vi "VI Tree.vi"   [LabVIEW 2017, in "Keithley 3390.lvlib"]
doc: "This is the instrument driver for the <INSTRUMENT NAME>. The VI Tree displays all the user-callable VIs of the instrument driver in an organized table."
uses:
  Keithley 3390.lvlib
  Configure/Configure Modulation (Amplitude).vi
  Configure/Low Level/Configure Voltage (Amplitude).vi
  Configure/Low Level/Configure Pulse (Period).vi
  Configure/Low Level/Configure Modulation Low Level (AM Depth).vi
  Configure/Configure Waveform (Sine).vi
panel:
  # "(c) 2008 Keithley Instruments, Inc..  ALL RIGHTS RESERVED."
  # "SEE DIAGRAM\nFOR VI TREE."
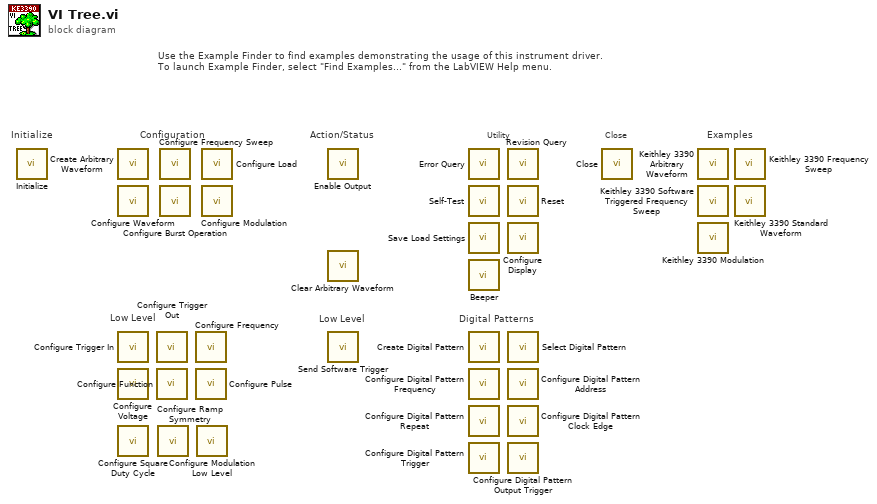
[diagram p0: block diagram]
diagram:
  # "Examples"
  # "Digital Patterns"
  # "Low Level"
  # "Low Level"
  # "Use the Example Finder to find examples demonstrating the usage of this instrument driver.\nTo launch Example Finder, select \"Find Examples...\" from the LabVIEW Help menu."
  # "Configuration"
  # "Utility"
  # "Action/Status"
  # "Close"
  # "Initialize"
  n1 = call "Initialize.vi"() -> ()  [unwired: 10 in, 2 out]
  n2 = call "Create Arbitrary Waveform.vi"() -> ()  [unwired: 10 in, 2 out]
  n3 = call-poly "Configure Waveform.vi"() -> ()  [unwired: 14 in, 2 out]
  n4 = call "Configure Trigger In.vi"() -> ()  [unwired: 10 in, 2 out]
  n5 = call-poly "Configure Voltage.vi"() -> ()  [unwired: 10 in, 2 out]
  n6 = call "Configure Square Duty Cycle.vi"() -> ()  [unwired: 10 in, 2 out]
  n7 = call "Configure Trigger Out.vi"() -> ()  [unwired: 10 in, 2 out]
  n8 = call "Configure Function.vi"() -> ()  [unwired: 10 in, 2 out]
  n9 = call "Configure Ramp Symmetry.vi"() -> ()  [unwired: 10 in, 2 out]
  n10 = call "Configure Frequency Sweep.vi"() -> ()  [unwired: 10 in, 2 out]
  n11 = call "Configure Burst Operation.vi"() -> ()  [unwired: 10 in, 2 out]
  n12 = call "Configure Frequency.vi"() -> ()  [unwired: 10 in, 2 out]
  n13 = call-poly "Configure Pulse.vi"() -> ()  [unwired: 10 in, 2 out]
  n14 = call-poly "Configure Modulation Low Level.vi"() -> ()  [unwired: 10 in, 2 out]
  n15 = call "Configure Load.vi"() -> ()  [unwired: 10 in, 2 out]
  n16 = call-poly "Configure Modulation.vi"() -> ()  [unwired: 10 in, 2 out]
  n17 = call "Enable Output.vi"() -> ()  [unwired: 10 in, 2 out]
  n18 = call "Clear Arbitrary Waveform.vi"() -> ()  [unwired: 10 in, 2 out]
  n19 = call "Send Software Trigger.vi"() -> ()  [unwired: 10 in, 2 out]
  n20 = call "Error Query.vi"() -> ()  [unwired: 8 in, 4 out]
  n21 = call "Self-Test.vi"() -> ()  [unwired: 8 in, 4 out]
  n22 = call "Save Load Settings.vi"() -> ()  [unwired: 14 in, 2 out]
  n23 = call "Beeper.vi"() -> ()  [unwired: 10 in, 2 out]
  n24 = call "Create Digital Pattern.vi"() -> ()  [unwired: 10 in, 2 out]
  n25 = call "Configure Digital Pattern Frequency.vi"() -> ()  [unwired: 10 in, 2 out]
  n26 = call "Configure Digital Pattern Repeat.vi"() -> ()  [unwired: 10 in, 2 out]
  n27 = call "Configure Digital Pattern Trigger.vi"() -> ()  [unwired: 10 in, 2 out]
  n28 = call "Revision Query.vi"() -> ()  [unwired: 8 in, 4 out]
  n29 = call "Reset.vi"() -> ()  [unwired: 10 in, 2 out]
  n30 = call "Configure Display.vi"() -> ()  [unwired: 14 in, 2 out]
  n31 = call "Select Digital Pattern.vi"() -> ()  [unwired: 10 in, 2 out]
  n32 = call "Configure Digital Pattern Address.vi"() -> ()  [unwired: 10 in, 2 out]
  n33 = call "Configure Digital Pattern Clock Edge.vi"() -> ()  [unwired: 10 in, 2 out]
  n34 = call "Configure Digital Pattern Output Trigger.vi"() -> ()  [unwired: 10 in, 2 out]
  n35 = call "Close.vi"() -> ()  [unwired: 11 in, 1 out]
  n36 = call "Keithley 3390 Arbitrary Waveform.vi"() -> ()  [unwired: 12 in]
  n37 = call "Keithley 3390 Software Triggered Frequency Sweep.vi"() -> ()  [unwired: 12 in]
  n38 = call "Keithley 3390 Modulation.vi"() -> ()  [unwired: 1 in]
  n39 = call "Keithley 3390 Frequency Sweep.vi"() -> ()  [unwired: 12 in]
  n40 = call "Keithley 3390 Standard Waveform.vi"() -> ()  [unwired: 12 in]
